vi "Array sorting.vi"(1 "index":dbl[](array[numeric]), 2 "Array In":dbl[][](array[numeric])) -> (0 "Array Out":dbl[][](array[numeric]))   [LabVIEW 2016]
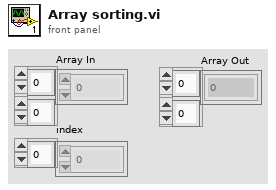
[diagram p1: front panel]
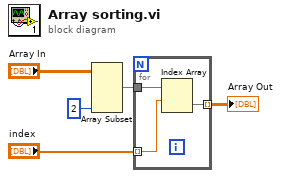
[diagram p0: block diagram]
diagram:
  n1 = Array Subset(array="Array In", length (col)=2 ("length")) -> (w1:dbl[][])  [unwired: 3 in]
  n2 = for {
    tunnel: w1 -> [w8]
    tunnel: [w7] -> w4 mode=indexing
    tunnel: "index" -> [w6] mode=indexing
    n3 = Index Array(array=w8, index (row)=w6) -> (element=w7:dbl[])  [unwired: 1 in]
  }
  "Array Out" <- w4
